vi "svc_Get SV Channel Info (variant).vi"(6 "channel index":i32, 8 "error in (no error)":errorcluster, 11 "attributes":variant) -> (0 "error out":errorcluster, 1 "unit label":string, 2 "channel info":T1={"sensor sensitivity"=1000.0, "engineering units"=1, "dB reference"=1.0, "custom label"="EU", "weighting filter"=0, "pregain"=0.0} {"pregain" format="%.2f"; "weighting filter" items=["Linear", "A-weighting", "B-weighting", "C-weighting", "ITU-R 468-4", "Dolby", "CCITT", "C-message", "Wb", "Wc", "Wd", "We", "Wf", "Wh", "Wj", "Wk", "Wm", "AES17 20 kHz lowpass", "AES17 40 kHz lowpass", "AES17 20 kHz highpass", "AES17 40 kHz highpass"]; "dB reference" format="%^.1e"; "engineering units" items=["custom..."=0, "V"=1, "A"=21, "C"=30, "pC"=31, "s"=32, "-"=29, "Pa"=2, "N"=20, "g"=3, "m/s^2"=4, "m/s"=5, "m"=6, "mm/s"=12, "mm"=13, "micron/s"=14, "micron"=15, "in/s^2"=7, "in/s"=8, "in"=9, "mil/s"=10, "mil"=11, "rad/s^2"=16, "rad/s"=17, "rad"=18, "deg/s^2"=26, "deg/s"=27, "deg"=28, "RPM"=22, "cycle/s^2"=23, "Hz"=24, "cycle"=25, "strain"=19]; "sensor sensitivity" format="%#_5f"}, 3 "dup attributes":variant, 5 "channel name":string, 7 "channel description":string)   [LabVIEW 2017]
uses:
  <vilib>/addons/_NISVFA/_Shared subVIs/Controls/svc_Channel Info.ctl
  <vilib>/addons/_NISVFA/_Shared subVIs/Controls/svc_Engineering Units Text Ring.ctl
  <vilib>/addons/_NISVFA/_Shared subVIs/Controls/svc_Weighting Filter Text Ring.ctl
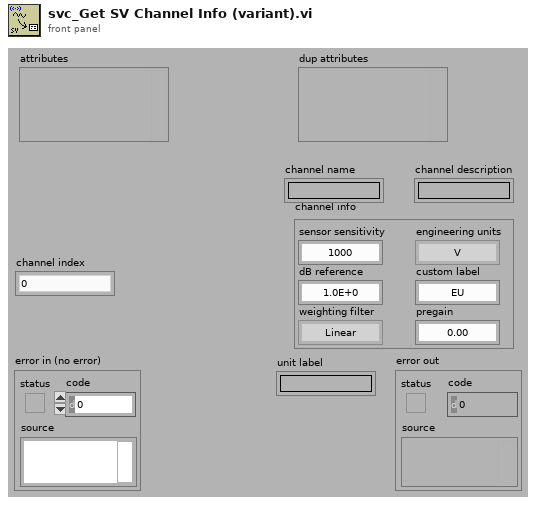
[diagram p1: front panel]
types:
  T1 = typedef "svc_Channel Info.ctl" = cluster{"sensor sensitivity":dbl, "engineering units":T2, "dB reference":dbl, "custom label":string, "weighting filter":T3, "pregain":dbl}
  T2 = typedef "svc_Engineering Units Text Ring.ctl" = u16
  T3 = typedef "svc_Weighting Filter Text Ring.ctl" = u16
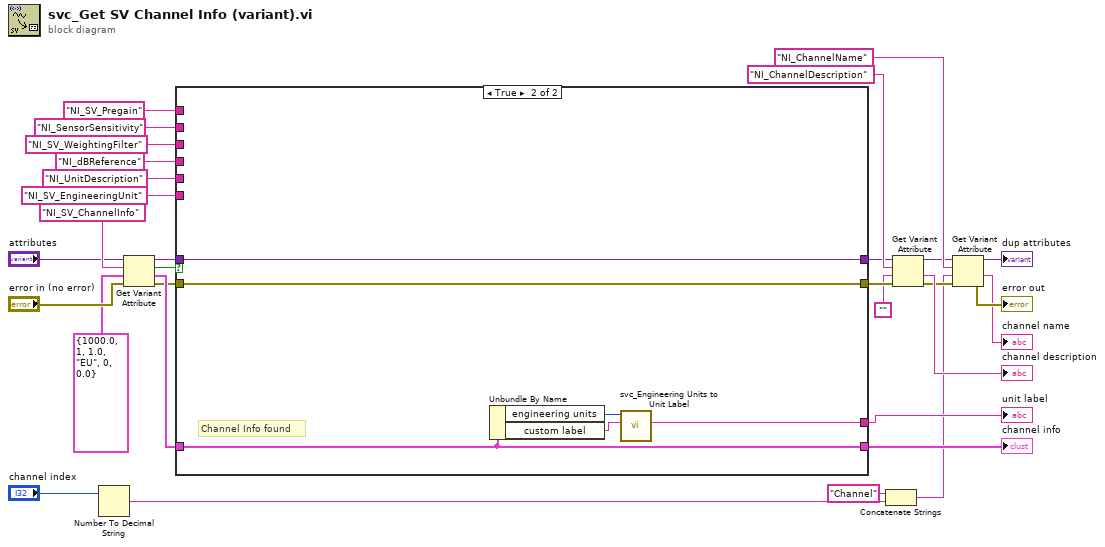
[diagram p0: block diagram]
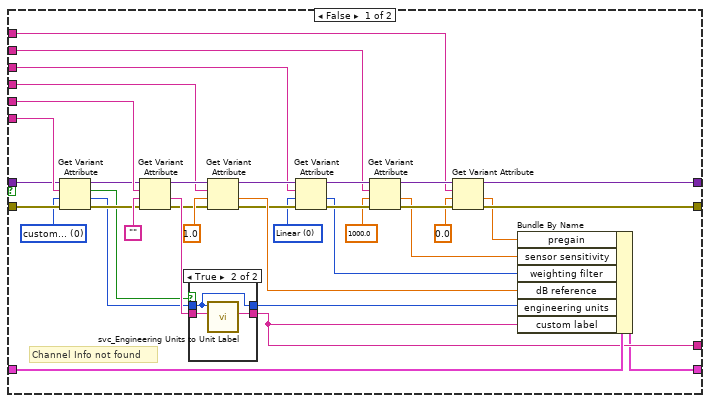
[diagram p2: hidden frame]
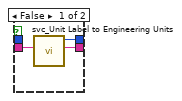
[diagram p3: hidden frame]
diagram:
  n1 = Number To Decimal String(number="channel index") -> (decimal integer string=w4:string)  [unwired: 1 in]
  n2 = Get Variant Attribute(Variant="attributes", name="NI_SV_ChannelInfo", default value (empty Variant)=T1 {"sensor sensitivity"=1000.0, "engineering units"=1, "dB reference"=1.0, "custom label"="EU", "weighting filter"=0, "pregain"=0.0} ("channel info"), error in="error in (no error)") -> (duplicate Variant=w22:variant, found=w23:bool, value=w21:T1, error out=w20:errorcluster)
  n3 = case shown="True" w23 {
    tunnel: w22 -> [w56 w79]
    tunnel: [w32 w78] -> w31
    tunnel: w21 -> [w65 w78]
    tunnel: w20 -> [w57 w80]
    tunnel: [w38 w80] -> w14
    tunnel: [w37 w79] -> w17
    tunnel: [w33 w75] -> w25
    tunnel: "NI_dBReference" ("name") -> [w60 _]
    tunnel: "NI_UnitDescription" ("name") -> [w59 _]
    tunnel: "NI_SV_EngineeringUnit" ("name") -> [w58 _]
    tunnel: "NI_SV_WeightingFilter" ("name") -> [w44 _]
    tunnel: "NI_SensorSensitivity" ("name") -> [w43 _]
    tunnel: "NI_SV_Pregain" ("name") -> [w42 _]
    frame False {
      w41 = T3 0 items=["Linear", "A-weighting", "B-weighting", "C-weighting", "ITU-R 468-4", "Dolby", "CCITT", "C-message"] ("weighting filter")
      w53 = T2 0 items=["custom..."=0, "V"=1, "A"=21, "Pa"=2, "N"=20, "g"=3, "m/s^2"=4, "m/s"=5, "m"=6, "mm/s"=12, "mm"=13, "micron/s"=14, "micron"=15, "in/s^2"=7, "in/s"=8, "in"=9, "mil/s"=10, "mil"=11, "rad/s^2"=16, "rad/s"=17, "rad"=18, "strain"=19] ("engineering units")
      # "Channel Info not found"
      n4 = Get Variant Attribute(Variant=w56, name=w58, default value (empty Variant)=w53, error in=w57) -> (duplicate Variant=w55:variant, found=w52:bool, value=w51:T2, error out=w54:errorcluster)
      n5 = Get Variant Attribute(Variant=w55, name=w59, default value (empty Variant)="" ("Empty String Constant"), error in=w54) -> (duplicate Variant=w62:variant, value=w67:string, error out=w61:errorcluster)  [unwired: 1 out]
      n6 = case shown="True" w52 {
        tunnel: w67 -> [w71 w73]
        tunnel: [w70 w72] -> w66
        tunnel: [w69 w74] -> w33
        tunnel: w51 -> [_ w72]
        frame False {
          n7 = call <vilib>:"svc_Unit Label to Engineering Units.vi"("unit label"=w71) -> ("unit label out"=w69:string, "engineering units"=w70:T2)  [unwired: 9 in]
        }
        frame True {
          n8 = call <vilib>:"svc_Engineering Units to Unit Label.vi"("custom label"=w73, "engineering units"=w72) -> ("unit label"=w74:string)  [unwired: 8 in, 1 out]
        }
      }
      n9 = Get Variant Attribute(Variant=w62, name=w60, default value (empty Variant)=1.0, error in=w61) -> (duplicate Variant=w50:variant, value=w63:dbl, error out=w49:errorcluster)  [unwired: 1 out]
      n10 = Get Variant Attribute(Variant=w50, name=w44, default value (empty Variant)=w41, error in=w49) -> (duplicate Variant=w47:variant, value=w35:T3, error out=w48:errorcluster)  [unwired: 1 out]
      n11 = Get Variant Attribute(Variant=w47, name=w43, default value (empty Variant)=1000.0 ("sensor sensitivity [mV/EU]"), error in=w48) -> (duplicate Variant=w45:variant, value=w36:dbl, error out=w46:errorcluster)  [unwired: 1 out]
      n12 = Get Variant Attribute(Variant=w45, name=w42, default value (empty Variant)=0.0 ("pregain [dB]"), error in=w46) -> (duplicate Variant=w37:variant, value=w34:dbl, error out=w38:errorcluster)  [unwired: 1 out]
      n13 = Bundle By Name(cluster=w65, "pregain"=w34, "sensor sensitivity"=w36, "weighting filter"=w35, "dB reference"=w63, "engineering units"=w66, "custom label"=w33) -> (w32:T1)
    }
    frame True {
      # "Channel Info found"
      n14 = Unbundle By Name(w78) -> ("engineering units"=w77:T2, "custom label"=w76:string)
      n15 = call <vilib>:"svc_Engineering Units to Unit Label.vi"("custom label"=w76, "engineering units"=w77) -> ("unit label"=w75:string)  [unwired: 8 in, 1 out]
    }
  }
  "channel info" <- w31
  "unit label" <- w25
  n16 = Concatenate Strings("Channel" ("string"), w4) -> (w3:string)
  n17 = Get Variant Attribute(Variant=w17, name="NI_ChannelDescription", default value (empty Variant)="" ("Empty String Constant"), error in=w14) -> (duplicate Variant=w16:variant, value=→"channel description":string, error out=w15:errorcluster)  [unwired: 1 out]
  n18 = Get Variant Attribute(Variant=w16, name="NI_ChannelName", default value (empty Variant)=w3, error in=w15) -> (duplicate Variant=→"dup attributes":variant, value=→"channel name":string, error out=→"error out":errorcluster)  [unwired: 1 out]
